vi "New RegReadExtLong Command.vi"(0 "RFFE RegReadExtLong Command in":refnum<class "RFFE RegReadExtLong Command.lvclass">, 5 "Slave Address":T2=12 format="%02x", 7 "Register Address":T1 format="%02x", 9 "Byte Count":i32=1, 11 "error in (no error)":errorcluster) -> (4 "RFFE RegReadExtLong Command out":refnum<class "RFFE RegReadExtLong Command.lvclass">, 15 "error out":errorcluster)   [LabVIEW 2018, in "MIPI RFFE API.lvlib" / "RFFE RegReadExtLong Command.lvclass"]
uses:
  RFFE RegReadExtLong Command.lvclass
  C:/Users/semoore/Projects/mipi-rffe-labview-oop/RegReadExt/RFFE RegReadExt Command.lvclass
  Slave Address.ctl
  Register Address.ctl
  RegReadExt/RFFE RegReadExt Command.lvclass
  MIPI RFFE API.lvlib
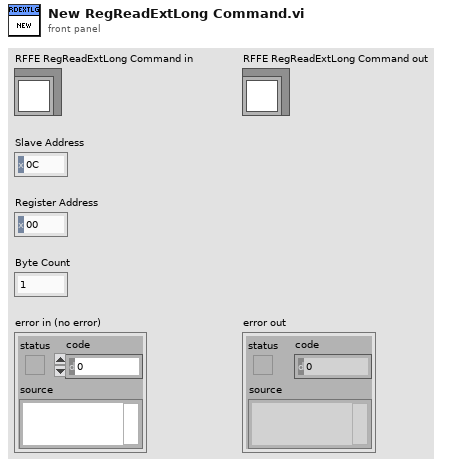
[diagram p1: front panel]
types:
  T1 = typedef "MIPI RFFE API.lvlib/Register Address.ctl" = u16
  T2 = typedef "MIPI RFFE API.lvlib/Slave Address.ctl" = u8
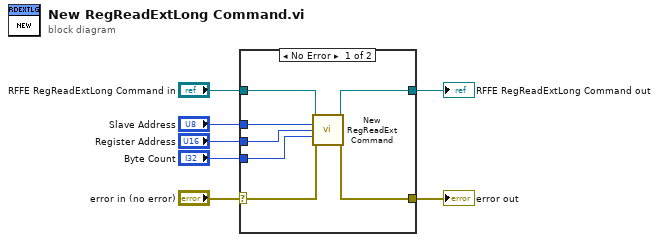
[diagram p0: block diagram]
diagram:
  n1 = case shown="No Error" "error in (no error)" {
    selector: "error in (no error)" -> [w12 w16]
    tunnel: [w11 w16] -> w6
    tunnel: [w14 w15] -> w4
    tunnel: "RFFE RegReadExtLong Command in" -> [w13 w15]
    tunnel: "Byte Count" -> [w10 _]
    tunnel: "Register Address" -> [w9 _]
    tunnel: "Slave Address" -> [w8 _]
    frame No Error {
      n2 = call "New RegReadExt Command.vi"("RFFE RegReadExt Command in"=w13, "Slave Address"=w8, "Register Address"=w9, "Byte Count"=w10, "error in (no error)"=w12) -> ("RFFE RegReadExt Command out"=w14:refnum<class "RFFE RegReadExtLong Command.lvclass">, "error out"=w11:errorcluster)  [unwired: 9 in]
    }
    frame Error {
    }
  }
  "error out" <- w6
  "RFFE RegReadExtLong Command out" <- w4
